vi "draw_overlay_2D.vi"(8 "error in (no error)":errorcluster, 10 "image in":refnum<class "Image.lvclass">, 11 "GenericTrajectory in":refnum<class "TrajectoryDL091126GenericVoxel.lvclass">) -> (0 "error out":errorcluster, 2 "image out":refnum<class "Image.lvclass">, 3 "GenericTrajectory out":refnum<class "TrajectoryDL091126GenericVoxel.lvclass">)   [LabVIEW 2010, in "TrajectoryDL091126GenericVoxel.lvclass"]
uses:
  TrajectoryDL091126GenericVoxel.lvclass
  common/classes/Image/Image/Image.lvclass
  common/classes/Image/Image/origin_type_enum.ctl
  common/enumerations/x_y_z_enumeration.ctl
  common/enumerations/functional_global_action_enum.ctl
  common/classes/ErrorController/ErrorController/class_data.vi
  common/classes/SpaceVector/SpaceVector/SpaceVector.lvclass
  common/classes/ErrorController/ErrorController/ErrorController.lvclass
panel:
  in  "colour":u32(colorbox)=16711680
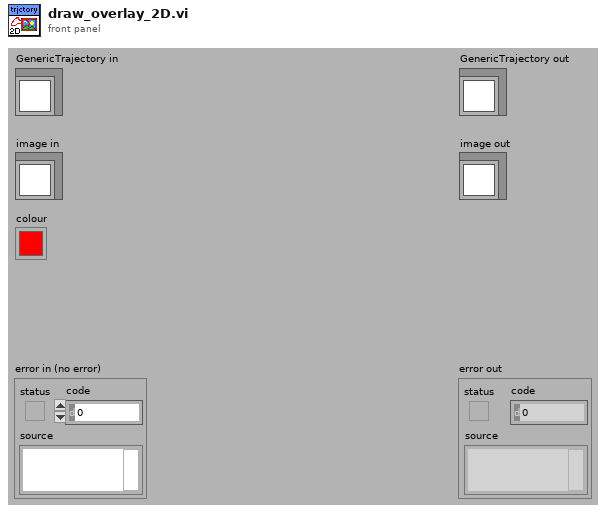
[diagram p1: front panel]
types:
  T1 = typedef "origin_type_enum.ctl" = enum16{"IMAQ origin", "middle of image"}
  T2 = typedef "x_y_z_enumeration.ctl" = enum16{"x", "y", "z"}
  T3 = typedef "functional_global_action_enum.ctl" = enum16{"get", "set", "reset"}
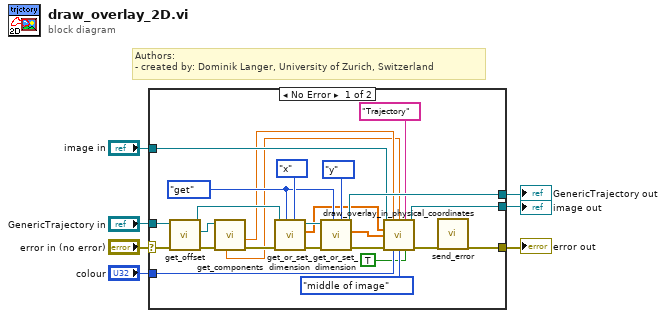
[diagram p0: block diagram]
diagram:
  # "Authors: \n- created by: Dominik Langer, University of Zurich, Switzerland"
  n1 = case shown="No Error" "error in (no error)" {
    selector: "error in (no error)" -> [w20 w34]
    tunnel: [w8 w34] -> w6
    tunnel: [w27 w33] -> w4
    tunnel: "GenericTrajectory in" -> [w19 w33]
    tunnel: "image in" -> [w26 _]
    tunnel: "colour" -> [w24 _]
    tunnel: [w21 _] -> w1
    frame No Error {
      w31 = functional_global_action_enum."get" ("action")
      n2 = call "get_offset.vi"("error in (no error)"=w20, "GenericTrajectory.lvclass in"=w19) -> ("error out"=w18:errorcluster, "SpaceVector.lvclass"=w15:refnum<class "SpaceVector.lvclass">, "GenericTrajectory.lvclass out"=w16:refnum<class "TrajectoryDL091126GenericVoxel.lvclass">)  [unwired: 7 in]
      n3 = call "get_components.vi"("error in (no error)"=w18, "SpaceVector in"=w15) -> ("error out"=w17:errorcluster, "x"=w14:dbl[unit], "y"=w13:dbl[unit])  [unwired: 4 in, 3 out]
      n4 = call-dynamic "get_or_set_dimension.vi"("dimension"=x_y_z_enumeration."x", "action"=w31, "error in (no error)"=w17, "GenericTrajectory in"=w16) -> ("error out"=w29:errorcluster, "pixel values out (single dimension)"=w23:dbl[unit][], "GenericTrajectory out"=w28:refnum<class "TrajectoryDL091126GenericVoxel.lvclass">)  [unwired: 5 in]
      n5 = call-dynamic "get_or_set_dimension.vi"("dimension"=x_y_z_enumeration."y", "action"=w31, "error in (no error)"=w29, "GenericTrajectory in"=w28) -> ("error out"=w25:errorcluster, "pixel values out (single dimension)"=w22:dbl[unit][], "GenericTrajectory out"=w27:refnum<class "TrajectoryDL091126GenericVoxel.lvclass">)  [unwired: 5 in]
      n6 = call "draw_overlay_in_physical_coordinates.vi"("Image in"=w26, "x offset"=w14, "y offset"=w13, "overlay group"="Trajectory", "x coordinates"=w23, "y coordinates"=w22, "error in (no error)"=w25, "colour"=w24, "origin"=origin_type_enum."middle of image", "clear previous overlay of this group?"=TRUE) -> ("Image out"=w21:refnum<class "Image.lvclass">, "error out"=w9:errorcluster)  [unwired: 4 in]
      n7 = call "send_error.vi"("error in (no error)"=w9) -> ("error out"=w8:errorcluster)  [unwired: 10 in]
    }
    frame Error {
    }
  }
  "error out" <- w6
  "GenericTrajectory out" <- w4
  "image out" <- w1
